vi "DRC91SettleT.vi"(0 "VISA Rsrc":refnum<visa-resource-name>="GPIB0::12::INSTR", 1 "Temp Ref":refnum<vi>, 2 "Stop Ref":refnum<vi>, 5 "SetPoint (K)":dbl, 7 "DevBand (K)":dbl=1.0, 9 "Channel":u16(ring) items=["A", "B"], 11 "error in":errorcluster, 12 "SettleTime(s)":u32=60, 13 "SampleRate(ms)":u32=2000) -> (4 "Données":dbl[](array[numeric]), 15 "error out":errorcluster)   [LabVIEW 2010]
doc: "Ce Vi interroge le contrôlleur de température pour la lecture en unités capteur des entrées spécifiées"
uses:
  <userlib>/GenProg/WritebyRefNum.vi
  <userlib>/GenProg/ReadbyRefBool.vi
panel:
  out "Reached":bool caption="Setpoint\nReached"
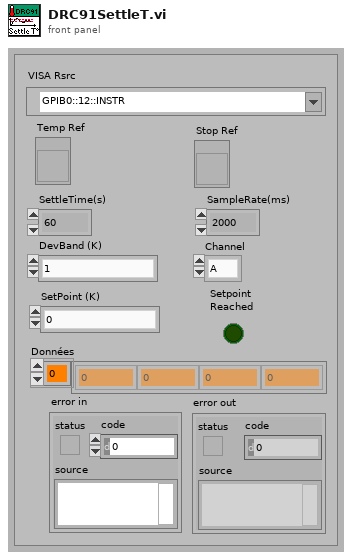
[diagram p1: front panel]
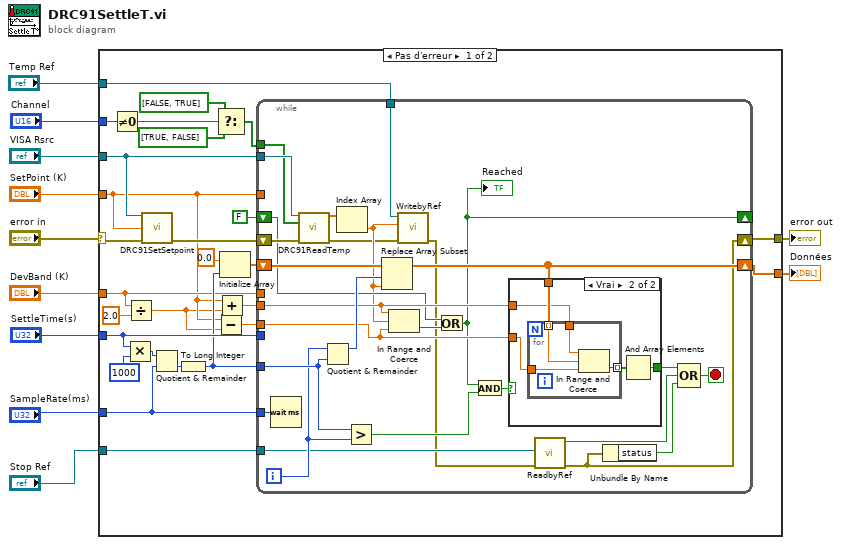
[diagram p0: block diagram]
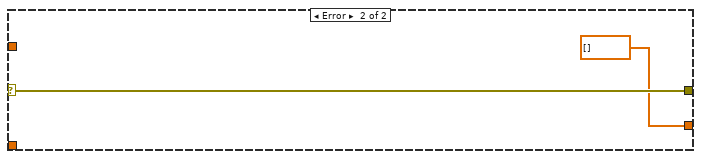
[diagram p3: hidden frame]
diagram:
  n1 = case shown="Pas d'erreur" "error in" {
    selector: "error in" -> [w36 w77]
    tunnel: [w38 w77] -> w11
    tunnel: "VISA Rsrc" -> [w37 _]
    tunnel: [w14 dbl[] []] -> w9
    tunnel: "SetPoint (K)" -> [w24 _]
    tunnel: "DevBand (K)" -> [w25 _]
    tunnel: "SampleRate(ms)" -> [w29 _]
    tunnel: "SettleTime(s)" -> [w34 _]
    tunnel: "Channel" -> [w19 _]
    tunnel: "Temp Ref" -> [w13 _]
    tunnel: "Stop Ref" -> [w12 _]
    frame No Error {
      n2 = Not Equal To 0?(x=w19) -> (x != 0?=w18:bool)
      n3 = Multiply(x=w34, y=u32 1000) -> (x*y=w30:u32)
      n4 = Divide(x=w25, y=2.0) -> (x/y=w23:dbl)
      n5 = call <userlib>:"DRC91SetSetpoint.vi"("VISA Rsrc"=w37, "SetPoint"=w24, "error in (no error)"=w36) -> ("error out"=w35:errorcluster)  [unwired: 12 in]
      n6 = Quotient & Remainder(x=w30, y=w29) -> (floor(x/y)=w28:u32)  [unwired: 1 out]
      n7 = To Long Integer(number=w28) -> (32bit integer=w27:i32)
      n8 = Select(t=bool[] [FALSE, TRUE], s=w18, f=bool[] [TRUE, FALSE]) -> (s? t:f=w15:bool[])
      n9 = Subtract(x=w24, y=w23) -> (x-y=w21:dbl)
      n10 = Add(x=w24, y=w23) -> (x+y=w22:dbl)
      n11 = Initialize Array(0.0 ("élément"), w27) -> (w31:dbl[])
      n12 = while {
        shift-right: [w39] -> w38
        shift-left: w35 -> [w65]
        tunnel: w24 -> [_]
        tunnel: w37 -> [w64]
        tunnel: w25 -> [_]
        shift-right: [w57] -> w14
        shift-left: w31 -> [w62]
        tunnel: w29 -> [w63]
        tunnel: w34 -> [_]
        tunnel: w27 -> [w60]
        tunnel: w22 -> [w56]
        tunnel: w21 -> [w55]
        shift-right: [w52] -> _
        shift-left: FALSE -> [w53]
        tunnel: w15 -> [w49]
        tunnel: w13 -> [w47]
        tunnel: w12 -> [w42]
        i -> [w59]
        stop <- w44 stop-if-true
        n13 = Wait (ms)(milliseconds to wait=w63) -> ()  [unwired: 1 out]
        n14 = call <userlib>:"DRC91ReadTemp.vi"("VISA Rsrc"=w64, "Activées"=w49, "error in"=w65) -> ("Données"=w61:dbl[], "error out"=w46:errorcluster)  [unwired: 10 in, 1 out]
        n15 = Quotient & Remainder(x=w59, y=w60) -> (x-y*floor(x/y)=w58:i32)  [unwired: 1 out]
        n16 = Index Array(array=w61) -> (element=w48:dbl)  [unwired: 1 in]
        n17 = Greater?(x=w60, y=w59) -> (0:w51:bool)
        n18 = Replace Array Subset(array=w62, new element=w48, index=w58) -> (w57:dbl[])
        n19 = In Range and Coerce(upper limit=w56, x=w48, lower limit=w55) -> (In Range?=w54:bool)  [unwired: 1 out]
        n20 = call-poly <userlib>:"WritebyRef.vi"("error in"=w46, "Valeur"=w48, "Control Ref"=w47) -> ("error out"=w40:errorcluster)  [unwired: 8 in]
        n21 = Or(x=w53, y=w54) -> (x .or. y?=w52:bool)
        "Reached" <- w52
        n22 = And(x=w52, y=w51) -> (x .and. y?=w50:bool)
        n23 = case shown="Vrai" w50 {
          selector: w50 -> [w66 _]
          tunnel: w57 -> [_ w71]
          tunnel: w56 -> [_ w70]
          tunnel: w55 -> [_ w69]
          tunnel: [w66 w67] -> w45
          frame False {
          }
          frame True {
            n24 = for {
              tunnel: w71 -> [w75] mode=indexing
              tunnel: w70 -> [w74]
              tunnel: w69 -> [w73]
              tunnel: [w72] -> w68 mode=indexing
              n25 = In Range and Coerce(upper limit=w74, x=w75, lower limit=w73) -> (In Range?=w72:bool)  [unwired: 1 out]
            }
            n26 = And Array Elements(Boolean array=w68) -> (logical AND=w67:bool)
          }
        }
        n27 = call-poly <userlib>:"ReadbyRef.vi"("error in"=w40, "Control Ref"=w42) -> ("error out"=w39:errorcluster, "Valeur"=w43:bool)  [unwired: 8 in]
        n28 = Unbundle By Name(w39) -> ("status"=w41:bool)
        n29 = Compound Arithmetic op=OR(w45, w43, w41) -> (w44:bool)
      }
    }
    frame Error {
    }
  }
  "error out" <- w11
  "Données" <- w9
